vi "Run.vi"(9 "API-Requests":T1, 10 "Broadcast-Enqueuers":T2, 11 "Actor in":refnum<class "Actor.lvclass">) -> (0 "error out":errorcluster, 3 "Actor out":refnum<class "Actor.lvclass">)   [LabVIEW 2018, in "Scripting.lvlib" / "Actor.lvclass"]
uses:
  Actor.lvclass
  Broadcast Enqueuers.ctl
  Did Initialize.ctl
  API-Requests.ctl
  Launch.ctl
  Stop.ctl
  Get State.ctl
  State.ctl
  Internal-Enqueuers.ctl
  Internal-Stop.ctl
  Internal-Error.ctl
types:
  T1 = typedef "Scripting.lvlib/Actor.lvclass/API-Requests.ctl" = refnum<event-registration>
  T2 = typedef "Scripting.lvlib/Actor.lvclass/Broadcast Enqueuers.ctl" = cluster{"Did Initialize":refnum<user-event>}
  T3 = typedef "Scripting.lvlib/Actor.lvclass/Internal-Enqueuers.ctl" = cluster{"Stop":refnum<user-event>, "Error":refnum<user-event>}
  T4 = cluster{"API-Requests":T1, "Internal-Launch":refnum<event-registration>, "Internal-Stop":refnum<event-registration>, "Internal-Stop":refnum<event-registration>}
  T5 = typedef "Scripting.lvlib/Actor.lvclass/Did Initialize.ctl" = cluster{"State":refnum<class "Actor.lvclass">}
  T6 = typedef "Scripting.lvlib/Actor.lvclass/State.ctl" = cluster{"Current State":refnum<class "Actor.lvclass">}
  T7 = typedef "Scripting.lvlib/Actor.lvclass/Internal-Stop.ctl" = cluster{"Type":enum16{"Normal", "Emergency"}}
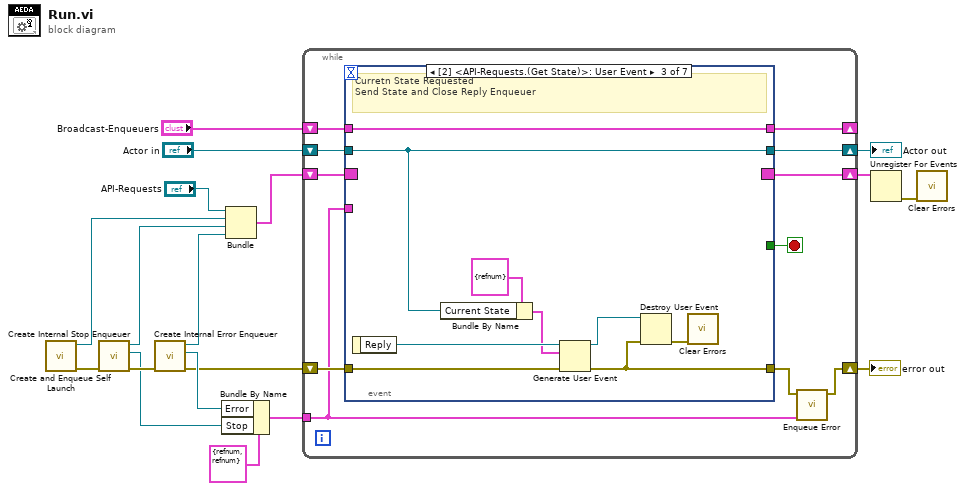
[diagram p0: block diagram]
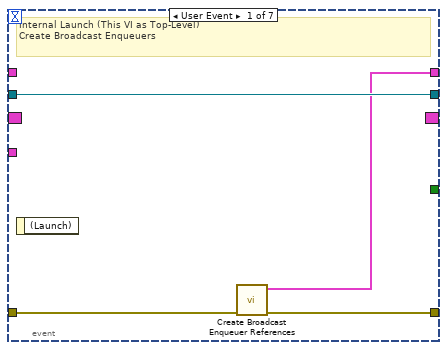
[diagram p2: hidden frame]
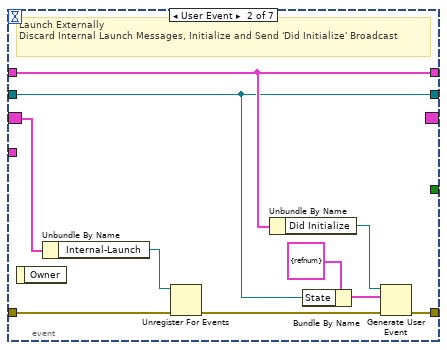
[diagram p3: hidden frame]
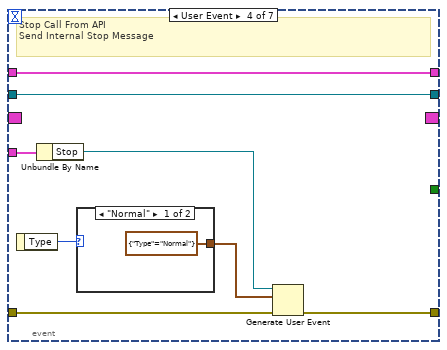
[diagram p4: hidden frame]
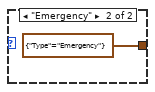
[diagram p5: hidden frame]
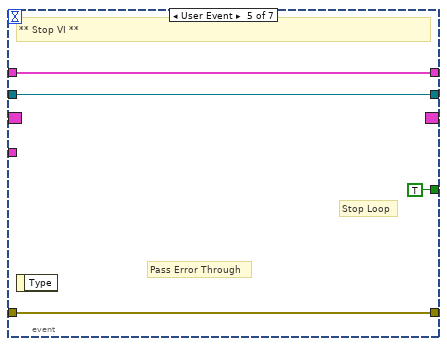
[diagram p6: hidden frame]
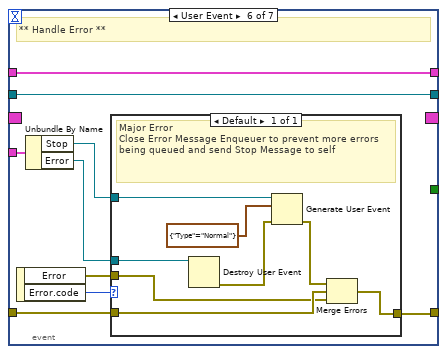
[diagram p7: hidden frame]
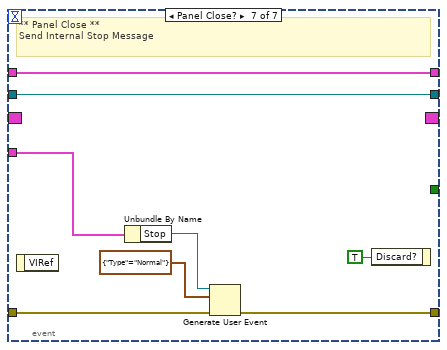
[diagram p8: hidden frame]
diagram:
  n1 = call "Create and Enqueue Self Launch.vi"() -> ("error out"=w13:errorcluster, "Internal-Launch"=w8:refnum<event-registration>)  [unwired: 10 in]
  n2 = call "Create Internal Stop Enqueuer.vi"("error in (no error)"=w13) -> ("error out"=w12:errorcluster, "Stop Enqueuer"=w10:refnum<user-event>, "Internal-Stop"=w7:refnum<event-registration>)  [unwired: 8 in]
  n3 = call "Create Internal Error Enqueuer.vi"("error in (no error)"=w12) -> ("error out"=w3:errorcluster, "Error Enqueuer"=w9:refnum<user-event>, "Internal-Stop"=w6:refnum<event-registration>)  [unwired: 8 in]
  n4 = Bundle By Name(cluster=T3 {"Stop"=refnum, "Error"=refnum} ("States"), "Error"=w9, "Stop"=w10) -> (w2:T3)
  n5 = Bundle("API-Requests"="API-Requests", "Internal-Launch"=w8, "Internal-Stop"=w7, "Internal-Stop"=w6) -> (w5:T4)  [unwired: 1 in]
  n6 = while {
    shift-right: [w27] -> w17
    shift-left: "Actor in" -> [w29]
    shift-right: [w23] -> w14
    shift-left: w3 -> [w28]
    shift-right: [w22] -> w4
    shift-left: w5 -> [w21]
    tunnel: w2 -> [w20]
    shift-right: [w19] -> _
    shift-left: "Broadcast-Enqueuers" -> [w25]
    stop <- w26 stop-if-true
    n7 = event shown="[2] <API-Requests.(Get State)>: User Event" {
      selector: w21 -> [_ w43 _ _ _ _ _]
      dyn-events: [_ _ _ _ _ _ _] -> w22
      timeout: _ -> [_ _ _ _ _ _ _]
      tunnel: w29 -> [w33 w34 w46 w60 w66 w75 w91]
      tunnel: w28 -> [w30 w41 w49 w59 w65 w74 w89]
      tunnel: [w33 w34 w46 w60 w66 w75 w91] -> w27
      tunnel: [w32 w38 w44 w58 w65 w72 w88] -> w24
      tunnel: [_ _ _ _ TRUE _ _] -> w26
      tunnel: w25 -> [_ w40 w52 w53 w63 w68 w84]
      tunnel: w20 -> [_ _ _ w55 _ w67 w86]
      tunnel: [w31 w40 w52 w53 w63 w68 w84] -> w19
      event User Event {
        # "Internal Launch (This VI as Top-Level)\nCreate Broadcast Enqueuers"
        n8 = event-data() -> ()  [unwired: 1 in, 1 out]
        n9 = call "Create Broadcast Enqueuer References.vi"("error in (no error)"=w30) -> ("error out"=w32:errorcluster, "Broadcasts"=w31:T2)  [unwired: 9 in]
      }
      event User Event {
        # "Launch Externally\nDiscard Internal Launch Messages, Initialize and Send 'Did Initialize' Broadcast"
        n10 = event-data() -> ()  [unwired: 1 in, 1 out]
        n11 = Unbundle By Name(w43) -> ("Internal-Launch"=w42:refnum<event-registration>)
        n12 = Unregister For Events(event registration refnum=w42, error in=w41) -> (error out=w39:errorcluster)
        n13 = Unbundle By Name(w40) -> ("Did Initialize"=w37:refnum<user-event>)
        n14 = Bundle By Name(cluster=T5 {"State"=refnum} ("event data"), "State"=w34) -> (w35:T5)
        n15 = Generate User Event(user event=w37, event data cluster=w35, error in=w39) -> (error out=w38:errorcluster)  [unwired: 1 in, 1 out]
      }
      event User Event {
        # "Curretn State Requested\nSend State and Close Reply Enqueuer"
        n16 = event-data() -> ("Reply"=w51:refnum<user-event>)  [unwired: 1 in]
        n17 = Bundle By Name(cluster=T6 {"Current State"=refnum} ("event data"), "Current State"=w46) -> (w47:T6)
        n18 = Generate User Event(user event=w51, event data cluster=w47, error in=w49) -> (user event out=w48:refnum<user-event>, error out=w44:errorcluster)  [unwired: 1 in]
        n19 = Destroy User Event(user event=w48, error in=w44) -> (error out=w45:errorcluster)
        n20 = call <vilib>:"Clear Errors.vi"("error in (no error)"=w45) -> ()  [unwired: 5 in, 2 out]
      }
      event User Event {
        # "Stop Call From API\nSend Internal Stop Message"
        n21 = event-data() -> ("Type"=w57:enum16{"Normal", "Emergency"})  [unwired: 1 in]
        n22 = Unbundle By Name(w55) -> ("Stop"=w54:refnum<user-event>)
        n23 = case shown="\"Normal\"" w57 {
          tunnel: [T7 {"Type"=enum."Normal"} ("event data") T7 {"Type"=enum."Emergency"} ("event data")] -> w56
          frame "Normal" {
          }
          frame "Emergency" {
          }
        }
        n24 = Generate User Event(user event=w54, event data cluster=w56, error in=w59) -> (error out=w58:errorcluster)  [unwired: 1 in, 1 out]
      }
      event User Event {
        # "Stop Loop"
        # "Pass Error Through"
        # "** Stop VI **"
        n25 = event-data() -> ()  [unwired: 1 in, 1 out]
      }
      event User Event {
        # "** Handle Error **"
        n26 = event-data() -> ("Error"=w69:errorcluster, "Error.code"=w70:i32)  [unwired: 1 in]
        n27 = Unbundle By Name(w67) -> ("Stop"=w73:refnum<user-event>, "Error"=w71:refnum<user-event>)
        n28 = case shown="Default" w70 {
          tunnel: w74 -> [w79]
          tunnel: w73 -> [w77]
          tunnel: [w82] -> w72
          tunnel: w71 -> [w76]
          tunnel: w69 -> [w78]
          frame Default {
            # "Major Error\nClose Error Message Enqueuer to prevent more errors being queued and send Stop Message to self"
            n29 = Destroy User Event(user event=w76) -> (error out=w83:errorcluster)  [unwired: 1 in]
            n30 = Generate User Event(user event=w77, event data cluster=T7 {"Type"=enum."Normal"} ("event data"), error in=w83) -> (error out=w81:errorcluster)  [unwired: 1 in, 1 out]
            n31 = Merge Errors(w81, w79, w78) -> (w82:errorcluster)
          }
        }
      }
      event Panel Close? {
        # "** Panel Close **\nSend Internal Stop Message"
        n32 = event-data() -> ()  [unwired: 1 in, 1 out]
        n33 = Unbundle By Name(w86) -> ("Stop"=w85:refnum<user-event>)
        n34 = Generate User Event(user event=w85, event data cluster=T7 {"Type"=enum."Normal"} ("event data"), error in=w89) -> (error out=w88:errorcluster)  [unwired: 1 in, 1 out]
        n35 = event-data("Discard?"=TRUE) -> ()  [unwired: 1 in, 1 out]
      }
    }
    n36 = call "Enqueue Error.vi"("Error-Enqueuer in"=w20, "error in (no error)"=w24) -> ("error out"=w23:errorcluster)  [unwired: 9 in]
  }
  "Actor out" <- w17
  "error out" <- w14
  n37 = Unregister For Events(event registration refnum=w4) -> (error out=w15:errorcluster)  [unwired: 1 in]
  n38 = call <vilib>:"Clear Errors.vi"("error in (no error)"=w15) -> ()  [unwired: 5 in, 2 out]
